vi "FPGA_Main.vi"() -> ()   [LabVIEW 2016]
uses:
  <vilib>/rvi/Emulation/niFpgaGetClockAttributes.vi
  <vilib>/rvi/Emulation/niFpgaSctlEmulationGetInTimedLoop.vi
  <vilib>/rvi/Emulation/niFpgaEmulationReportErrorSimple.vi
  <vilib>/rvi/eio/common/nirviEmuTemplateMethod_errors.vi
  <vilib>/rvi/Emulation/niFpgaCriticalErrorInLSC.vi
  <vilib>/eio/EIONode/EIONode.xnode
panel:
  in  "Servo2HighTime":u32(slide) scale=0.0..2000.0
  in  "Servo1HighTime":u32(slide) scale=0.0..2000.0
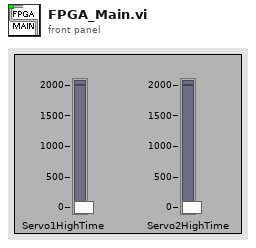
[diagram p1: front panel]
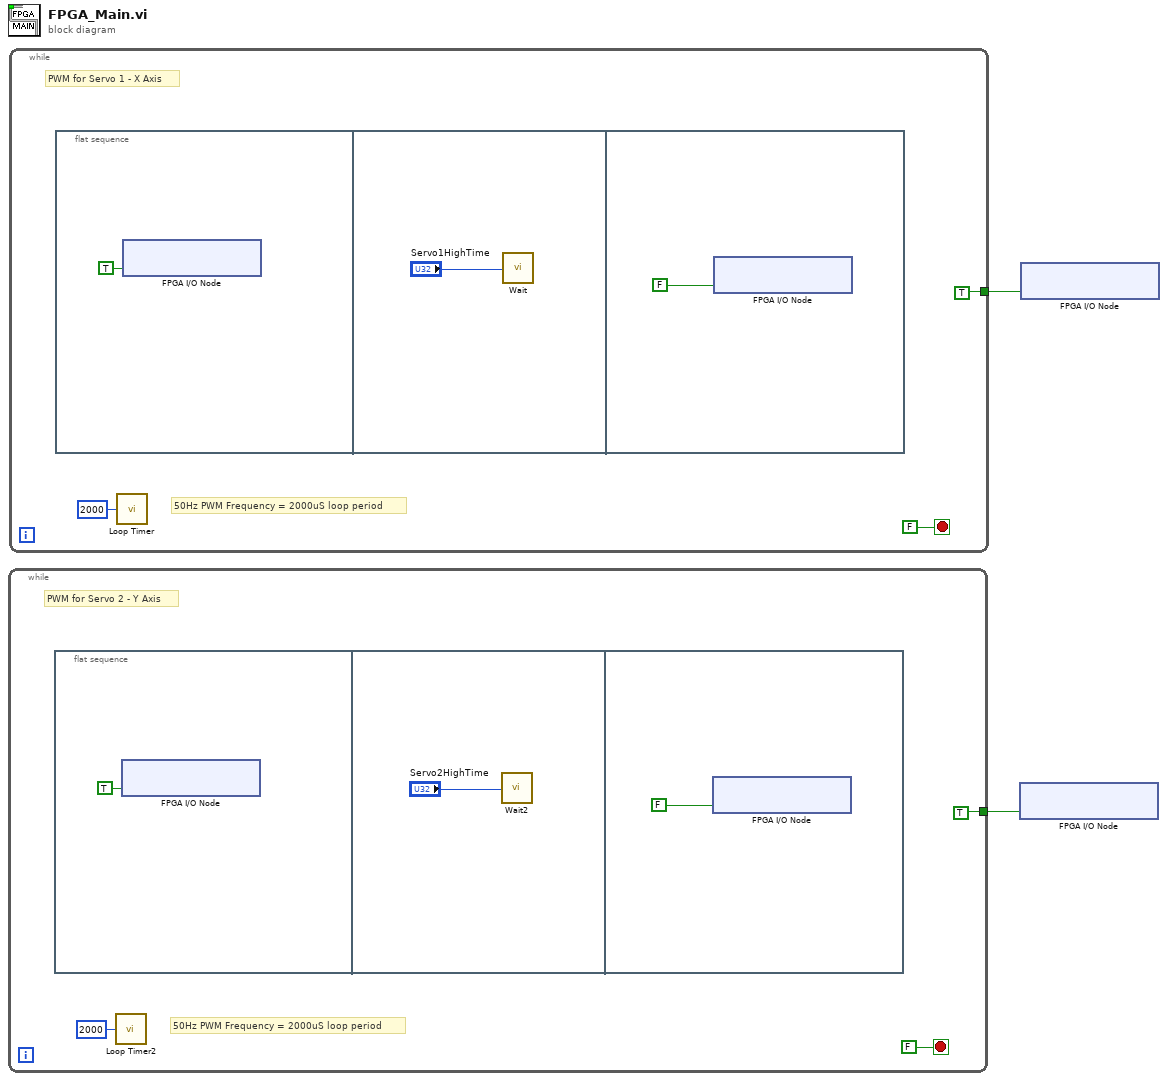
[diagram p0: block diagram]
diagram:
  n1 = while {
    tunnel: [TRUE ("ConnectorC/DIO3")] -> w1
    stop <- FALSE stop-if-true
    # "PWM for Servo 2 - Y Axis"
    # "50Hz PWM Frequency = 2000uS loop period"
    n2 = flat-sequence {
      frame #0 {
        n3 = xnode "FPGA I/O Node"("ConnectorC/DIO7"=TRUE ("ConnectorA/DIO3")) -> ()  [unwired: 1 in, 1 out]
      }
      frame #1 {
        n4 = call "Wait2"("Count(uSec)"="Servo2HighTime") -> ()  [unwired: 1 out]
      }
      frame #2 {
        n5 = xnode "FPGA I/O Node"("ConnectorC/DIO7"=FALSE ("ConnectorA/DIO3")) -> ()  [unwired: 1 in, 1 out]
      }
    }
    n6 = call "Loop Timer2"("Count(uSec)"=u32 2000) -> ()  [unwired: 1 out]
  }
  n7 = while {
    tunnel: [TRUE ("ConnectorC/DIO3")] -> w2
    stop <- FALSE stop-if-true
    # "PWM for Servo 1 - X Axis"
    # "50Hz PWM Frequency = 2000uS loop period"
    n8 = flat-sequence {
      frame #0 {
        n9 = xnode "FPGA I/O Node"("ConnectorC/DIO3"=TRUE ("ConnectorA/DIO3")) -> ()  [unwired: 1 in, 1 out]
      }
      frame #1 {
        n10 = call "Wait"("Count(uSec)"="Servo1HighTime") -> ()  [unwired: 1 out]
      }
      frame #2 {
        n11 = xnode "FPGA I/O Node"("ConnectorC/DIO3"=FALSE ("ConnectorA/DIO3")) -> ()  [unwired: 1 in, 1 out]
      }
    }
    n12 = call "Loop Timer"("Count(uSec)"=u32 2000) -> ()  [unwired: 1 out]
  }
  n13 = xnode "FPGA I/O Node"("ConnectorC/DIO7"=w1) -> ()  [unwired: 1 in, 1 out]
  n14 = xnode "FPGA I/O Node"("ConnectorC/DIO3"=w2) -> ()  [unwired: 1 in, 1 out]
